vi "Flywheel_Hardware_Loop.vi"   [LabVIEW 2020]
uses:
  <vilib>/Rock Robotics/WPI/ThirdParty/Phoenix-LabVIEW/Motor Controller/Controls/CTRE_Phoenix_MotorControl_ControlMode.ctl
  Flywheel_Hardware_Globals.vi
  Globals/Flywheel_Globals.vi
types:
  T1 = typedef "WPI_MotorControlDeviceRef.ctl" = cluster{"DeviceStatus":errorcluster, "Type":T2, "PWM":cluster{"PWM Channel":T3, "DeadBand":T4}, "CAN":cluster{"Device Number":u8, "SetOutput VI Ref":variant, "GetOutput VI Ref":variant, "Enable VI Ref":variant, "Disable VI Ref":variant, "Data":variant}, "Invert":bool, "DIO PWM":cluster{"PWM \"Enable\" Channel":T3, "DIOChannel":T5, "PWM Rate":dbl}}
  T2 = typedef "WPI_MotorControlType.ctl" = enum16{"PWM", "CAN", "DIO PWM"}
  T3 = typedef "FPGA_DIOPWMChannel.ctl" = enum8{"PWM 0", "PWM 1", "PWM 2", "PWM 3", "PWM 4", "PWM 5", "PWM 6", "PWM 7", "PWM 8", "PWM 9", "PWM MXP 0", "PWM MXP 1", "PWM MXP 2", "PWM MXP 3", "PWM MXP 4", "PWM MXP 5", "PWM MXP 6", "PWM MXP 7", "PWM MXP 8", "PWM MXP 9", "Invalid"}
  T4 = typedef "WPI_PWMDeadband.ctl" = cluster{"Name":string, "maxPositivePwm":i32, "minPositivePwm":i32, "centerPwm":i32, "maxNegativePwm":i32, "minNegativePwm":i32, "angularRange":u16}
  T5 = typedef "FPGA_DIOChannel.ctl" = enum8{"DIO 0", "DIO 1", "DIO 2", "DIO 3", "DIO 4", "DIO 5", "DIO 6", "DIO 7", "DIO 8", "DIO 9", "DIO MXP 0", "DIO MXP 1", "DIO MXP 2", "DIO MXP 3", "DIO MXP 4", "DIO MXP 5", "DIO MXP 6", "DIO MXP 7", "DIO MXP 8", "DIO MXP 9", "DIO MXP 10", "DIO MXP 11", "DIO MXP 12", "DIO MXP 13", "DIO MXP 14", "DIO MXP 15", "SPI Port CS1", "SPI Port CS2", "SPI Port CS3", "SPI Port MISO", "SPI Port MOSI", "Invalid"}
  T6 = typedef "Basic_Motor_Modes.ctl" = enum16{"Percent_Voltage", "Speed_Control", "Position_Control", "Current"}
  T7 = typedef "CTRE_Phoenix_MotorControl_ControlMode.ctl" = u16
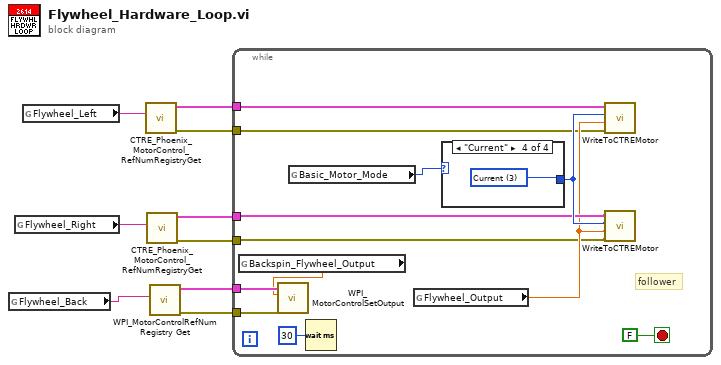
[diagram p0: block diagram]
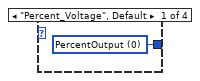
[diagram p2: hidden frame]
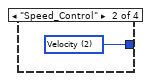
[diagram p3: hidden frame]
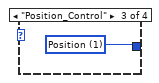
[diagram p4: hidden frame]
diagram:
  n1 = global read "Flywheel_Hardware_Globals.vi" "Flywheel_Back"() -> (w3:string)
  n2 = global read "Flywheel_Hardware_Globals.vi" "Flywheel_Right"() -> (w9:string)
  n3 = global read "Flywheel_Hardware_Globals.vi" "Flywheel_Left"() -> (w8:string)
  n4 = call <vilib>:"CTRE_Phoenix_MotorControl_RefNumRegistryGet.vi"("refnum name"=w8) -> ("error out"=w6:errorcluster, "PhoenixMotorControlDevRef"=w7:T1)  [unwired: 9 in]
  n5 = call <vilib>:"CTRE_Phoenix_MotorControl_RefNumRegistryGet.vi"("refnum name"=w9) -> ("error out"=w4:errorcluster, "PhoenixMotorControlDevRef"=w5:T1)  [unwired: 9 in]
  n6 = call <vilib>:"WPI_MotorControlRefNum Registry Get.vi"("refnum name"=w3) -> ("error out"=w1:errorcluster, "MotorControlDevRef"=w2:T1)  [unwired: 9 in]
  n7 = while {
    tunnel: w7 -> [w18]
    tunnel: w6 -> [w14]
    tunnel: w5 -> [w16]
    tunnel: w4 -> [w13]
    tunnel: w2 -> [w12]
    tunnel: w1 -> [w11]
    stop <- FALSE stop-if-true
    # "follower"
    n8 = global read "Flywheel_Globals.vi" "Backspin_Flywheel_Output"() -> (w10:dbl)
    n9 = call <vilib>:"WPI_MotorControlSetOutput.vi"("error in (no error)"=w11, "Output"=w10, "MotorControlDevRef"=w12) -> ()  [unwired: 6 in, 3 out]
    n10 = global read "Flywheel_Globals.vi" "Basic_Motor_Mode"() -> (w21:T6)
    n11 = Wait (ms)(milliseconds to wait=u32 30) -> ()  [unwired: 1 out]
    n12 = global read "Flywheel_Globals.vi" "Flywheel_Output"() -> (w15:dbl)
    n13 = case shown="\"Current\"" w21 {
      tunnel: [w22 w23 w24 w25] -> w17
      frame "Percent_Voltage", Default {
        w22 = T7 0 items=["PercentOutput"=0, "Position"=1, "Velocity"=2, "Current"=3, "Follower"=5, "MotionProfile"=6, "MotionMagic"=7, "MotionProfileArc"=10, "Disabled"=15] ("Control Mode")
      }
      frame "Speed_Control" {
        w23 = T7 2 items=["PercentOutput"=0, "Position"=1, "Velocity"=2, "Current"=3, "Follower"=5, "MotionProfile"=6, "MotionMagic"=7, "MotionProfileArc"=10, "Disabled"=15] ("Control Mode")
      }
      frame "Position_Control" {
        w24 = T7 1 items=["PercentOutput"=0, "Position"=1, "Velocity"=2, "Current"=3, "Follower"=5, "MotionProfile"=6, "MotionMagic"=7, "MotionProfileArc"=10, "Disabled"=15] ("Control Mode")
      }
      frame "Current" {
        w25 = T7 3 items=["PercentOutput"=0, "Position"=1, "Velocity"=2, "Current"=3, "Follower"=5, "MotionProfile"=6, "MotionMagic"=7, "MotionProfileArc"=10, "Disabled"=15] ("Control Mode")
      }
    }
    n14 = call "WriteToCTREMotor.vi"("error in (no error)"=w14, "Motor_Value"=w15, "Control Mode"=w17, "PhoenixMotorControlDevRef"=w18) -> ()  [unwired: 8 in]
    n15 = call "WriteToCTREMotor.vi"("error in (no error)"=w13, "Motor_Value"=w15, "Control Mode"=w17, "PhoenixMotorControlDevRef"=w16) -> ()  [unwired: 8 in]
  }
